vi "UI.vi"(8 "error in (no error)":errorcluster, 11 "Session  Name":string) -> (0 "error out":errorcluster)   [LabVIEW 2018, in "Process Bar.lvclass"]
uses:
  Process Bar.lvclass
panel:
  out "Horizontal Progress Bar":u8(slide) scale=0.0..100.0
  out "SYSTEM STATUS":string
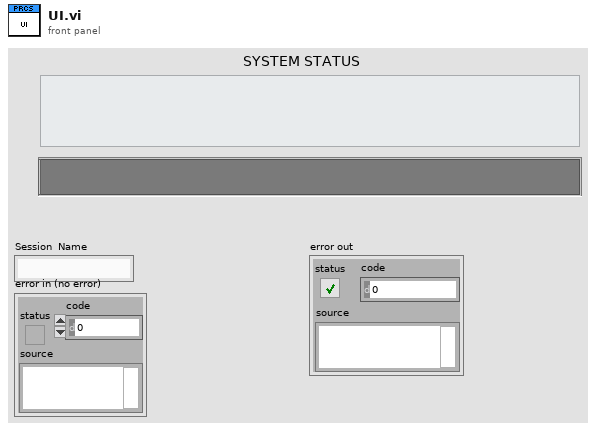
[diagram p1: front panel]
types:
  T1 = typedef "Process Bar.lvclass/Session Handle.ctl" = refnum<data-value>
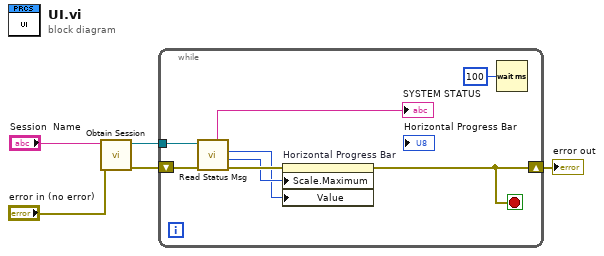
[diagram p0: block diagram]
diagram:
  n1 = call "Obtain Session.vi"("error in (no error)"="error in (no error)", "Session  Name ()"="Session  Name") -> ("error out"=w4:errorcluster, "Session Handle"=w5:T1)  [unwired: 8 in]
  n2 = while {
    tunnel: w5 -> [w12]
    shift-right: [w8] -> w3
    shift-left: w4 -> [w11]
    stop <- w8 stop-if-true
    n3 = call "Read Status Msg.vi"("error in (no error)"=w11, "Session Handle in"=w12) -> ("error out"=w9:errorcluster, "Process Max"=w7:u16, "Process Bar"=w6:u8, "Status Msg"=→"SYSTEM STATUS":string)  [unwired: 5 in, 1 out]
    n4 = property on="Horizontal Progress Bar" class="Slide (strict)"(error in=w9, "Scale.Maximum"=w7, "Value"=w6) -> (error out=w8:errorcluster)  [unwired: 1 in, 1 out]
    n5 = Wait (ms)(milliseconds to wait=u32 100) -> ()  [unwired: 1 out]
  }
  "error out" <- w3
